vi "Get Input Script.vi"(8 "error in (no error)":errorcluster, 10 "RxData Out":u16[](array[numeric]) format="%02x", 11 "Device Type":i32) -> (0 "error out":errorcluster, 1 "Force Targets":dbl[](array[numeric]), 2 "GAINC Reprogram?":string, 3 "GAINC Value":string, 4 "Variable Dwell":dbl[](array[numeric]), 5 "PID":T1, 6 "Input Script Letter":string)   [LabVIEW 2013]
uses:
  <vilib>/Utility/NIReport.llb/NI_report.lvclass
  InputScript states.ctl
  <vilib>/Utility/NIReport.llb/Excel/NI_Excel.lvclass
  <vilib>/addons/_office/NI_ReportGenerationToolkit.lvlib
  <vilib>/addons/_office/excel.llb/Excel Get Data (str).vi
  <vilib>/addons/_office/excel.llb/Excel Get Data ([dbl]).vi
  <vilib>/addons/_office/excel.llb/Excel Easy Table (str).vi
  <vilib>/addons/_office/excel.llb/Excel Get Data ([str]).vi
panel:
  out "output array":string[][](array[string])
  in  "State":T2
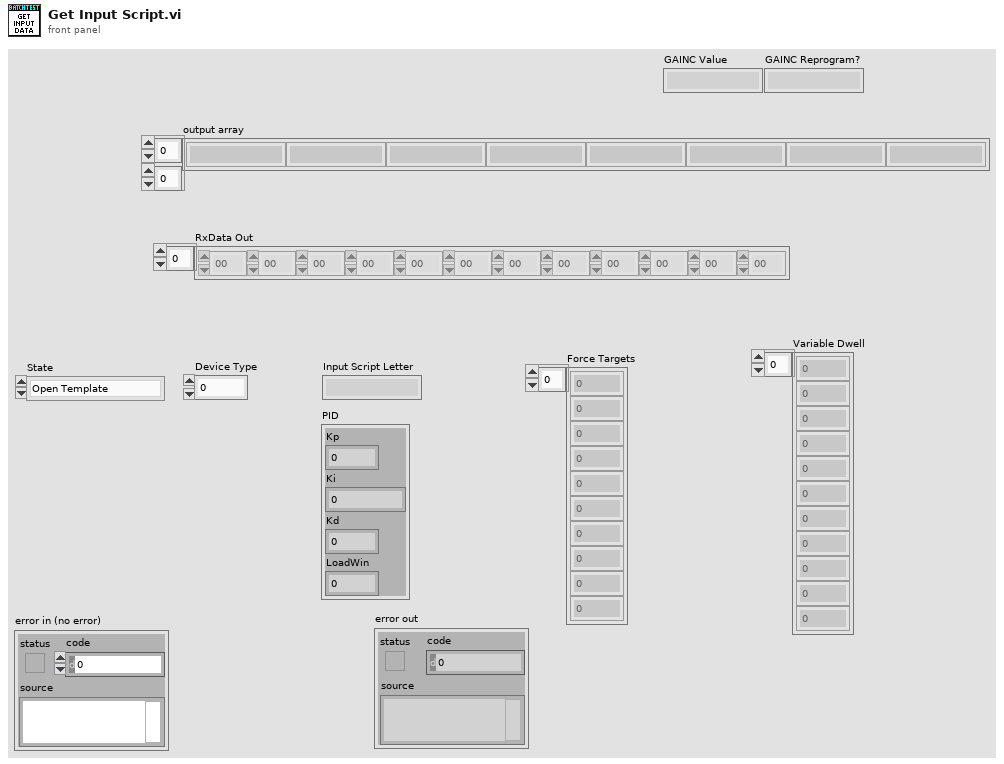
[diagram p1: front panel]
types:
  T1 = cluster{"Kp":dbl, "Ki":dbl, "Kd":dbl, "LoadWin":dbl}
  T2 = typedef "InputScript states.ctl" = enum16{"Open Template", "Setup parameters", "Read Input Script", "Close Template"}
  T3 = enum16{"Standard Report", "HTML", "Word", "Excel"}
  T4 = cluster{"[0]":dbl, "[1]":dbl, "[2]":dbl, "[3]":dbl, "[4]":dbl, "[5]":dbl, "[6]":dbl, "[7]":dbl, "[8]":dbl}
  T5 = cluster{"[0]":dbl, "[1]":dbl, "[2]":dbl, "[3]":dbl}
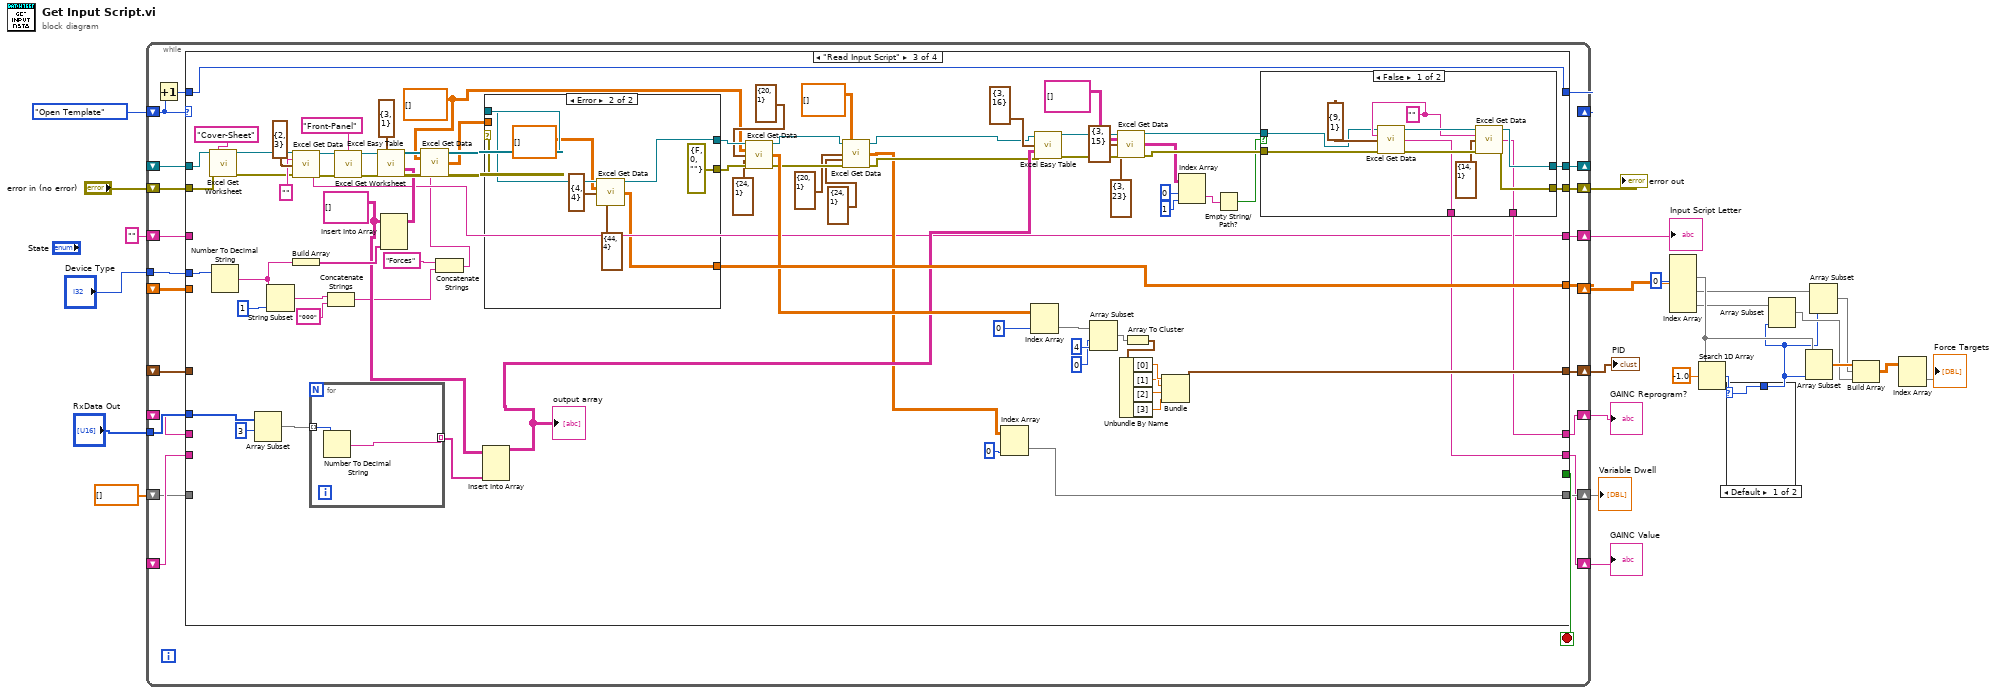
[diagram p0: block diagram]
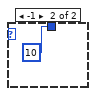
[diagram p2: hidden frame]
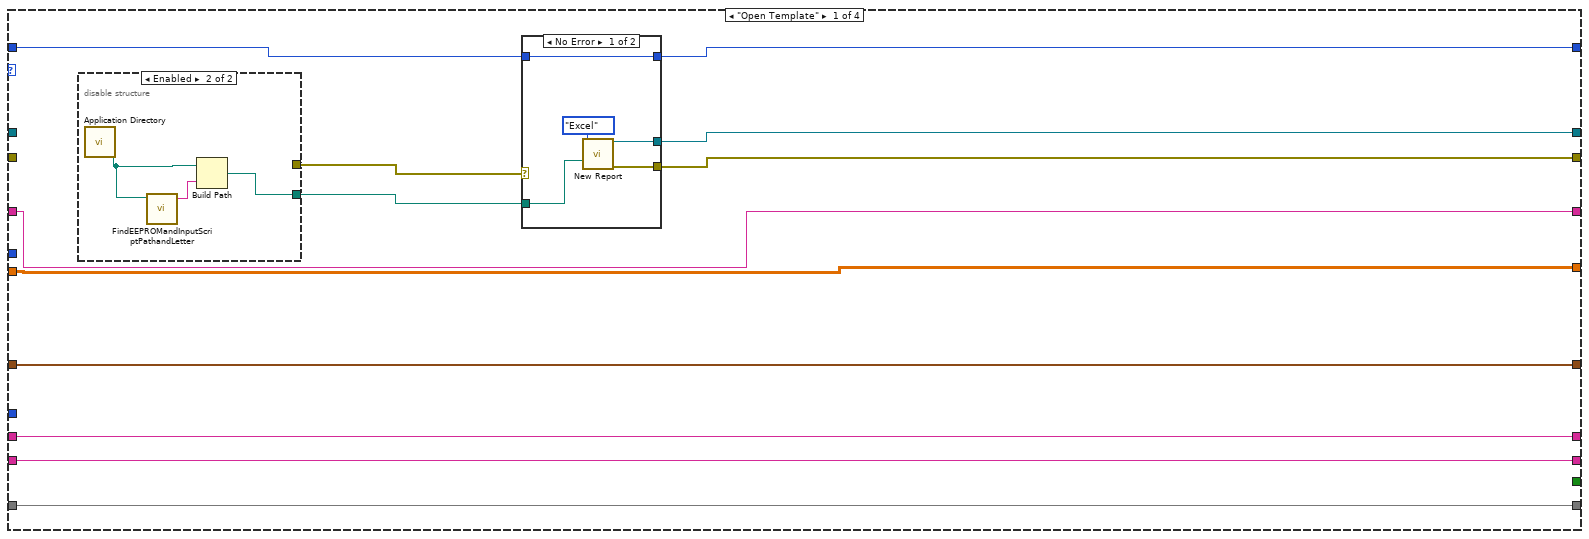
[diagram p3: hidden frame]
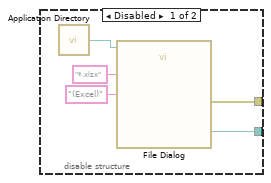
[diagram p4: hidden frame]
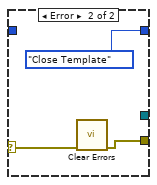
[diagram p5: hidden frame]
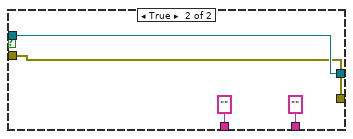
[diagram p7: hidden frame]
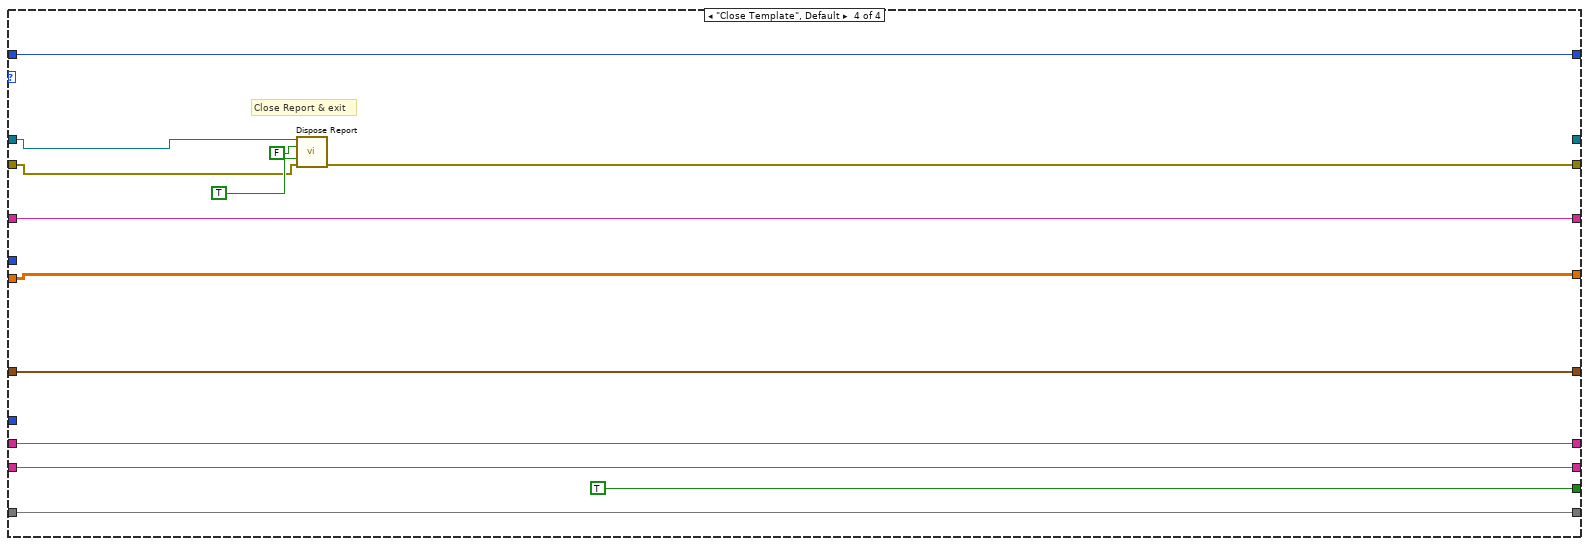
[diagram p9: hidden frame]
diagram:
  n1 = while {
    shift-right: [w46] -> _
    shift-left: _ -> [w45]
    shift-right: [w44] -> w23
    shift-left: "error in (no error)" -> [w43]
    shift-right: [w40] -> _
    shift-left: InputScript_states."Open Template" -> [w42]
    shift-right: [w39] -> w22
    shift-left: "" ("Input Script Letter") -> [w38]
    tunnel: "Device Type" -> [w37]
    shift-right: [w36] -> w8
    shift-left: _ -> [w35]
    shift-right: [w33] -> w6
    shift-left: _ -> [w34]
    tunnel: "RxData Out" -> [w32]
    shift-right: [w27] -> w4
    shift-left: _ -> [w31]
    shift-right: [w26] -> w3
    shift-left: _ -> [w30]
    shift-right: [w29] -> w1
    shift-left: dbl[] [] ("data") -> [w28]
    stop <- w47 stop-if-true
    n2 = Increment(x=w42) -> (x+1=w41:T2)
    n3 = case shown="\"Read Input Script\"" w42 {
      tunnel: [_ _ _ TRUE] -> w47
      tunnel: [w59 w84 w121 _] -> w46
      tunnel: w45 -> [_ w84 w155 w194]
      tunnel: [w58 w83 w120 w204] -> w44
      tunnel: w43 -> [_ w83 w154 w193]
      tunnel: w41 -> [w55 w82 w165 w202]
      tunnel: [w54 w82 w165 w202] -> w40
      tunnel: [w53 w81 w87 w201] -> w39
      tunnel: w38 -> [w53 w81 _ w201]
      tunnel: w37 -> [_ _ w116 _]
      tunnel: [w52 w80 w146 w200] -> w36
      tunnel: w35 -> [w52 w80 _ w200]
      tunnel: [w51 w76 w90 w199] -> w29
      tunnel: w28 -> [w51 w76 _ w199]
      tunnel: [w50 w79 w129 w198] -> w33
      tunnel: w34 -> [w50 w79 _ w198]
      tunnel: w32 -> [_ _ w128 _]
      tunnel: [w48 w77 w119 w196] -> w26
      tunnel: [w49 w78 w118 w197] -> w27
      tunnel: w31 -> [w49 w78 _ w197]
      tunnel: w30 -> [w48 w77 _ w196]
      frame "Open Template" {
        n4 = disable-structure shown="Enabled" {
          disable-tunnel: [w61 w67] -> w57
          disable-tunnel: [w60 _] -> w56
          frame Disabled {
            n5 = call <vilib>:"Application Directory.vi"() -> ("Application Directory"=w62:path)
            n6 = call "File Dialog"("start path"=w62, "pattern (all files)"="*.xlsx", "pattern label"="(Excel)") -> ("selected path"=w61:path, "error out"=w60:errorcluster)  [unwired: 9 in, 2 out]
          }
          frame Enabled {
            n7 = call <vilib>:"Application Directory.vi"() -> ("Application Directory"=w66:path)
            n8 = call "FindEEPROMandInputScriptPathandLetter.vi"("path"=w66) -> ("EEPROM File"=w65:string)  [unwired: 3 in, 3 out]
            n9 = Build Path(base path=w66, name or relative path=w65) -> (appended path=w67:path)
          }
        }
        n10 = case shown="No Error" w56 {
          selector: w56 -> [_ w75]
          tunnel: [w71 _] -> w59
          tunnel: [w70 w74] -> w58
          tunnel: w57 -> [w69 _]
          tunnel: w55 -> [w68 _]
          tunnel: [w68 InputScript_states."Close Template"] -> w54
          frame No Error {
            n11 = call <vilib>:"New Report.vi"("report type"=T3."Excel", "template (empty)"=w69) -> ("report out"=w71:refnum<class "NI_report.lvclass">, "error out"=w70:errorcluster)  [unwired: 12 in]
          }
          frame Error {
            n12 = call <vilib>:"Clear Errors.vi"("error in (no error)"=w75) -> ("error out"=w74:errorcluster)  [unwired: 5 in, 1 out]
          }
        }
      }
      frame "Setup parameters" {
      }
      frame "Read Input Script" {
        w98 = dbl[][] [] ("data type")
        w124 = string[][] [] ("array")
        n13 = call <vilib>:"Excel Get Worksheet.vi"("report in"=w155, "error in (no error)"=w154, "name (\"\")"="Cover-Sheet" ("name (\"\")")) -> ("report out"=w153:refnum<class "NI_report.lvclass">, "error out"=w152:errorcluster)  [unwired: 11 in]
        n14 = Number To Decimal String(number=w116) -> (decimal integer string=w115:string)  [unwired: 1 in]
        n15 = Array Subset(array=w128, index=3) -> (w125:u16[])  [unwired: 1 in]
        n16 = String Subset(string=w115, length (rest)=1 ("length (rest)")) -> (substring=w113:string)  [unwired: 1 in]
        n17 = call-poly <vilib>:"Excel Get Data.vi"("report in"=w153, "data type"="", "start (0, 0)"=cluster{"start row":i32, "start column":i32} {"start row"=2, "start column"=3}, "error in (no error)"=w152) -> ("report out"=w151:refnum<class "NI_report.lvclass">, "data"=w87:string, "error out"=w150:errorcluster)  [unwired: 9 in]
        n18 = Build Array(w115) -> (w160:string[])
        n19 = for {
          tunnel: w125 -> [w182] mode=indexing
          tunnel: [w181] -> w123 mode=indexing
          n20 = Number To Decimal String(number=w182) -> (decimal integer string=w181:string)  [unwired: 1 in]
        }
        n21 = Concatenate Strings(w113, "000" ("string")) -> (w111:string)
        n22 = call <vilib>:"Excel Get Worksheet.vi"("report in"=w151, "error in (no error)"=w150, "name (\"\")"="Front-Panel" ("name (\"\")")) -> ("report out"=w162:refnum<class "NI_report.lvclass">, "error out"=w161:errorcluster)  [unwired: 11 in]
        n23 = Insert Into Array(array=w124, new element=w160) -> (w159:string[][])  [unwired: 2 in]
        n24 = call-poly <vilib>:"Excel Easy Table.vi"("report in"=w162, "start (0, 0)"=cluster{"row":i32, "column":i32} {"row"=3, "column"=1}, "text data"=w159, "error in (no error)"=w161) -> ("report out"=w149:refnum<class "NI_report.lvclass">, "error out"=w148:errorcluster)  [unwired: 7 in, 3 out]
        n25 = Concatenate Strings("Forces" ("string"), w111) -> (w86:string)
        n26 = call-poly <vilib>:"Excel Get Data.vi"("report in"=w149, "data type"=w98, "error in (no error)"=w148, "name (\"\")"=w86) -> ("report out"=w145:refnum<class "NI_report.lvclass">, "data"=w85:dbl[][], "error out"=w147:errorcluster)  [unwired: 9 in]
        n27 = Insert Into Array(array=w124, new element=w123) -> (w122:string[][])  [unwired: 2 in]
        "output array" <- w122
        n28 = case shown="Error" w147 {
          selector: w147 -> [w184 _]
          tunnel: w85 -> [w185 _]
          tunnel: [w185 w187] -> w146
          tunnel: [w184 errorcluster {"status"=FALSE, "code"=0, "source"=""} ("error IO")] -> w143
          tunnel: w145 -> [w183 w191]
          tunnel: [w183 w190] -> w144
          frame No Error {
          }
          frame Error {
            n29 = call-poly <vilib>:"Excel Get Data.vi"("report in"=w191, "data type"=dbl[][] [], "start (-1, -1)"=cluster{"row":i32, "column":i32} {"row"=4, "column"=4}, "end (-1, -1)"=cluster{"row":i32, "column":i32} {"row"=44, "column"=4}) -> ("report out"=w190:refnum<class "NI_report.lvclass">, "data"=w187:dbl[][])  [unwired: 9 in, 1 out]
          }
        }
        n30 = call-poly <vilib>:"Excel Get Data.vi"("report in"=w144, "data type"=w98, "start (-1, -1)"=cluster{"row":i32, "column":i32} {"row"=20, "column"=1}, "end (-1, -1)"=cluster{"row":i32, "column":i32} {"row"=24, "column"=1}, "error in (no error)"=w143) -> ("report out"=w96:refnum<class "NI_report.lvclass">, "data"=w140:dbl[][], "error out"=w95:errorcluster)  [unwired: 8 in]
        n31 = call-poly <vilib>:"Excel Get Data.vi"("report in"=w96, "data type"=dbl[][] [], "start (-1, -1)"=cluster{"row":i32, "column":i32} {"row"=20, "column"=1}, "end (-1, -1)"=cluster{"row":i32, "column":i32} {"row"=24, "column"=1}, "error in (no error)"=w95) -> ("report out"=w93:refnum<class "NI_report.lvclass">, "data"=w91:dbl[][], "error out"=w94:errorcluster)  [unwired: 8 in]
        n32 = Index Array(array=w91, index (col)=0 ("index (row)")) -> (element=w90:dbl[])  [unwired: 1 in]
        n33 = Index Array(array=w140, index (col)=0 ("index (row)")) -> (element=w138:dbl[])  [unwired: 1 in]
        n34 = call-poly <vilib>:"Excel Easy Table.vi"("report in"=w93, "start (0, 0)"=cluster{"row":i32, "column":i32} {"row"=3, "column"=16}, "text data"=w122, "error in (no error)"=w94) -> ("report out"=w110:refnum<class "NI_report.lvclass">, "error out"=w109:errorcluster)  [unwired: 7 in, 3 out]
        n35 = Array Subset(array=w138, index=0, length=4) -> (w136:dbl[])
        n36 = call-poly <vilib>:"Excel Get Data.vi"("report in"=w110, "data type"=string[][] [], "start (-1, -1)"=cluster{"row":i32, "column":i32} {"row"=3, "column"=15}, "end (-1, -1)"=cluster{"row":i32, "column":i32} {"row"=3, "column"=23}, "error in (no error)"=w109) -> ("report out"=w108:refnum<class "NI_report.lvclass">, "data"=w104:string[][], "error out"=w107:errorcluster)  [unwired: 8 in]
        n37 = Array To Cluster(array=w136) -> (cluster=w134:T4)
        n38 = Unbundle By Name(w134) -> ("[0]"=w133:dbl, "[1]"=w132:dbl, "[2]"=w131:dbl, "[3]"=w130:dbl)
        n39 = Bundle("[0]"=w133, "[1]"=w132, "[2]"=w131, "[3]"=w130) -> (w129:T5)  [unwired: 1 in]
        n40 = Index Array(array=w104, index (row)=0, index (col)=1 ("disabled index (col)")) -> (element=w100:string)
        n41 = Empty String/Path?(string/path=w100) -> (empty?=w99:bool)
        n42 = case shown="False" w99 {
          tunnel: [w174 w180] -> w121
          tunnel: [w173 w179] -> w120
          tunnel: [w171 "" ("data")] -> w119
          tunnel: [w170 "" ("data")] -> w118
          tunnel: w108 -> [w167 w180]
          tunnel: w107 -> [w166 w179]
          frame False {
            w168 = ""
            n43 = call-poly <vilib>:"Excel Get Data.vi"("report in"=w167, "data type"=w168, "start (0, 0)"=cluster{"row":i32, "column":i32} {"row"=9, "column"=1}, "error in (no error)"=w166) -> ("report out"=w176:refnum<class "NI_report.lvclass">, "data"=w171:string, "error out"=w175:errorcluster)  [unwired: 9 in]
            n44 = call-poly <vilib>:"Excel Get Data.vi"("report in"=w176, "data type"=w168, "start (0, 0)"=cluster{"start row":i32, "start column":i32} {"start row"=14, "start column"=1}, "error in (no error)"=w175) -> ("report out"=w174:refnum<class "NI_report.lvclass">, "data"=w170:string, "error out"=w173:errorcluster)  [unwired: 9 in]
          }
          frame True {
          }
        }
      }
      frame "Close Template", Default {
        # "Close Report & exit"
        n45 = call-dynamic "Dispose Report.vi"("report in"=w194, "wait until printing completed? (T)"=FALSE, "save changes? (F)"=TRUE, "error in (no error)"=w193) -> ("error out"=w204:errorcluster)  [unwired: 11 in]
      }
    }
  }
  "error out" <- w23
  "Input Script Letter" <- w22
  "PID" <- w6
  "GAINC Reprogram?" <- w4
  "GAINC Value" <- w3
  "Variable Dwell" <- w1
  n46 = Index Array(array=w8, index (col) #1=0 ("index (row)")) -> (element #1=w16:dbl[], element #2=w14:dbl[], element #3=w13:dbl[])  [unwired: 5 in]
  n47 = Search 1D Array(1D array=w16, element=-1.0) -> (index of element=w17:i32)  [unwired: 1 in]
  n48 = case shown="Default" w17 {
    selector: w17 -> [w206 _]
    tunnel: [w206 10 ("index of element")] -> w10
    frame Default {
    }
    frame -1 {
    }
  }
  n49 = Array Subset(array=w13, length=w10) -> (w11:dbl[])  [unwired: 1 in]
  n50 = Array Subset(array=w16, length=w10) -> (w15:dbl[])  [unwired: 1 in]
  n51 = Array Subset(array=w14, length=w10) -> (w12:dbl[])  [unwired: 1 in]
  n52 = Build Array(w15, w12, w11) -> (w9:dbl[][])
  n53 = Index Array(array=w9) -> (element=→"Force Targets":dbl[])  [unwired: 2 in]
